vi "Reset myRIO.vi"(8 "error in (no error)":errorcluster) -> (0 "error out":errorcluster)   [LabVIEW 2021, in "Utilities.lvlib"]
doc: "Resets the FPGA target and all the I/O channels."
uses:
  <vilib>/myRIO/Instrument Drivers/Utilities/Utilities.lvlib
  <vilib>/myRIO/Common/Instrument Driver Framework/Utilities/typedefs/FPGA Ref Manager Action Enum.ctl
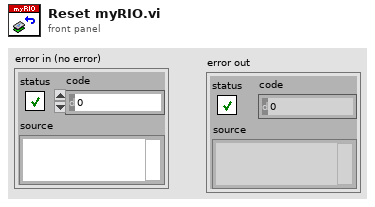
[diagram p1: front panel]
types:
  T1 = typedef "FPGA Ref Manager Action Enum.ctl" = enum16{"Get", "Set", "Reset"}
  T2 = typedef "Generic FPGA Reference.ctl" = refnum<k20>
  T3 = typedef "Block Write Resource.ctl" = refnum<vi>
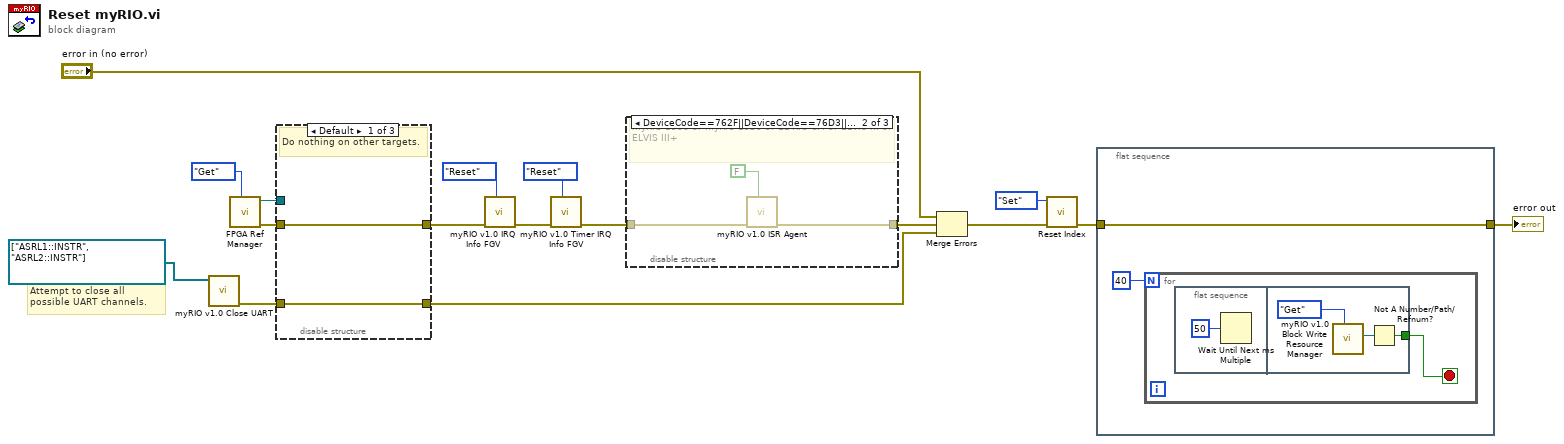
[diagram p0: block diagram]
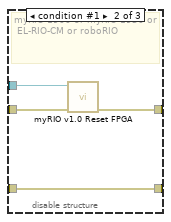
[diagram p2: hidden frame]
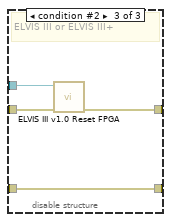
[diagram p3: hidden frame]
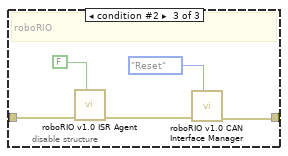
[diagram p5: hidden frame]
diagram:
  # "Attempt to close all possible UART channels."
  n1 = call <vilib>:"myRIO v1.0 Close UART.vi"("VISA resource array"=refnum<visa-resource-name>[] ["ASRL1::INSTR", "ASRL2::INSTR"]) -> ("error out"=w7:errorcluster)  [unwired: 10 in]
  n2 = call <vilib>:"FPGA Ref Manager.vi"("Action"=FPGA_Ref_Manager_Action_Enum."Get" ("Ref Counter Action Enum")) -> ("error out"=w8:errorcluster, "Generic FPGA Reference out"=w10:T2)  [unwired: 8 in]
  n3 = disable-structure shown="Default" {
    disable-tunnel: w10 -> [_ w21 w25]
    disable-tunnel: [w19 w23 w27] -> w9
    disable-tunnel: w8 -> [w19 w22 w26]
    disable-tunnel: w7 -> [w18 w20 w24]
    disable-tunnel: [w18 w20 w24] -> w6
    frame condition #0 (active) {
      # "Do nothing on other targets."
    }
    frame condition #1 {
      # "myRIO-1900 or myRIO-1950 or\n EL-RIO-CM or roboRIO"
      n4 = call <vilib>:"myRIO v1.0 Reset FPGA.vi"("error in (no error)"=w22, "Generic FPGA Reference in"=w21) -> ("error out"=w23:errorcluster)  [unwired: 8 in, 1 out]
    }
    frame condition #2 {
      # "ELVIS III or ELVIS III+"
      n5 = call <vilib>:"ELVIS III v1.0 Reset FPGA.vi"("error in (no error)"=w26, "Generic FPGA Reference in"=w25) -> ("error out"=w27:errorcluster)  [unwired: 8 in, 1 out]
    }
  }
  n6 = call <vilib>:"myRIO v1.0 IRQ Info FGV.vi"("Action"=FPGA_Ref_Manager_Action_Enum."Reset", "error in (no error)"=w9) -> ("error out"=w13:errorcluster)  [unwired: 8 in, 1 out]
  n7 = call <vilib>:"myRIO v1.0 Timer IRQ Info FGV.vi"("Action"=FPGA_Ref_Manager_Action_Enum."Reset", "error in (no error)"=w13) -> ("error out"=w12:errorcluster)  [unwired: 8 in, 1 out]
  n8 = disable-structure shown="DeviceCode==762F||DeviceCode==76D3||DeviceCode==7885||DeviceCode==7928||DeviceCode==793C" {
    disable-tunnel: w12 -> [w28 w30 w35]
    disable-tunnel: [w28 w29 w33] -> w11
    frame condition #0 (active) {
      # "Do nothing on other targets."
    }
    frame condition #1 {
      # "myRIO-1900 or myRIO-1950 or EL-RIO-CM or ELVIS III or ELVIS III+"
      n9 = call <vilib>:"myRIO v1.0 ISR Agent.vi"("Run?"=FALSE, "error in (no error)"=w30) -> ("error out"=w29:errorcluster)  [unwired: 9 in]
    }
    frame condition #2 {
      # "roboRIO"
      n10 = call <vilib>:"roboRIO v1.0 ISR Agent.vi"("Run?"=FALSE, "error in (no error)"=w35) -> ("error out"=w32:errorcluster)  [unwired: 9 in]
      n11 = call <vilib>:"roboRIO v1.0 CAN Interface Manager.vi"("Action"=FPGA_Ref_Manager_Action_Enum."Reset", "error in (no error)"=w32) -> ("error out"=w33:errorcluster)  [unwired: 8 in, 1 out]
    }
  }
  n12 = Merge Errors("error in (no error)", w11, w6) -> (w4:errorcluster)
  n13 = call <vilib>:"Reset Index.vi"("error in (no error)"=w4, "Action"=enum16{"Get", "Set"}."Set") -> ("error out"=w2:errorcluster)  [unwired: 8 in, 1 out]
  n14 = flat-sequence {
    tunnel: w2 -> [w38]
    tunnel: [w38] -> w1
    frame #0 {
      n15 = for {
        N: 40 -> [_]
        stop <- w39 stop-if-true
        n16 = flat-sequence {
          tunnel: [w41] -> w39
          frame #0 {
            n17 = Wait Until Next ms Multiple(millisecond multiple=u32 50 ("milliseconds to wait")) -> ()  [unwired: 1 out]
          }
          frame #1 {
            n18 = call <vilib>:"myRIO v1.0 Block Write Resource Manager.vi"("Action"=enum16{"Get", "Set", "Reset"}."Get") -> ("Resource Data Out"=w42:T3)  [unwired: 10 in]
            n19 = Not A Number/Path/Refnum?(number/path/refnum=w42) -> (NaN/Path/Refnum?=w41:bool)
          }
        }
      }
    }
  }
  "error out" <- w1
